vi "LOERN_Initialize.vi"() -> (14 "Fatal Error Out":T3, 15 "State Out":T1={"Inputs"=1, "SelectedIndex"=1, "ClassInfo"=[]})   [LabVIEW 2016, in "LV Object Event Registration Node.xnode"]
uses:
  LV Object Event Registration Node.xnode
  <vilib>/XNodeSupport/XNodeErrorCluster.ctl
  LOERN_State.ctl
  LOERN_ClassInfo.ctl
  <vilib>/XNodeSupport/NI_XNodeSupport.lvlib
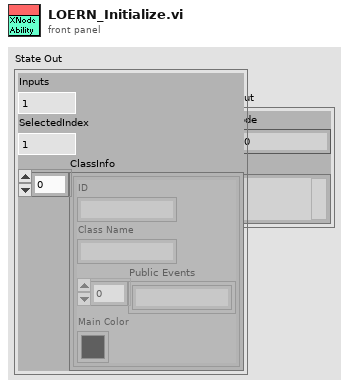
[diagram p1: front panel]
types:
  T1 = typedef "LV Object Event Registration Node.xnode/LOERN_State.ctl" = cluster{"Inputs":u16, "SelectedIndex":i16, "ClassInfo":T2[]}
  T2 = typedef "LV Object Event Registration Node.xnode/LOERN_ClassInfo.ctl" = cluster{"ID":string, "Class Name":string, "Public Events":string[], "Main Color":u32}
  T3 = typedef "NI_XNodeSupport.lvlib/XNodeErrorCluster.ctl" = errorcluster
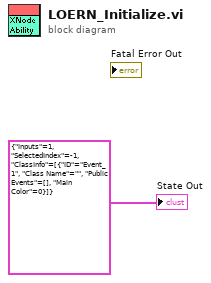
[diagram p0: block diagram]
diagram:
  "State Out" <- T1 {"Inputs"=1, "SelectedIndex"=-1, "ClassInfo"=[{"ID"="Event_1", "Class Name"="", "Public Events"=[], "Main Color"=0}]} ("State Out")
